vi "AM.vi"() -> ()   [LabVIEW 2015]
uses:
  <vilib>/express/express analysis/Spectral/Block/exnSpectralBlock spectral measurements RMS poly.vi
  <vilib>/express/express analysis/Spectral/Block/exnSpectralBlock spectral measurements RMS DDT.vi
  <vilib>/express/express analysis/Spectral/XNode/ExpressSpectralMeasurementsBlockNode.xnode
panel:
  out "Waveform Graph":dynamicdata(graph)
  out "Message":dynamicdata(graph)
  in  "Carrier Amp":dbl(slide) scale=0.0..10.0
  in  "Message Frequency":dbl(slide) scale=100.0..200.0
  in  "Carrier Frequency":dbl(slide) scale=0.0..10000.0
  out "AM":dynamicdata(graph)
  in  "stop":bool
  in  "m":dbl(slide) scale=0.0..2.0
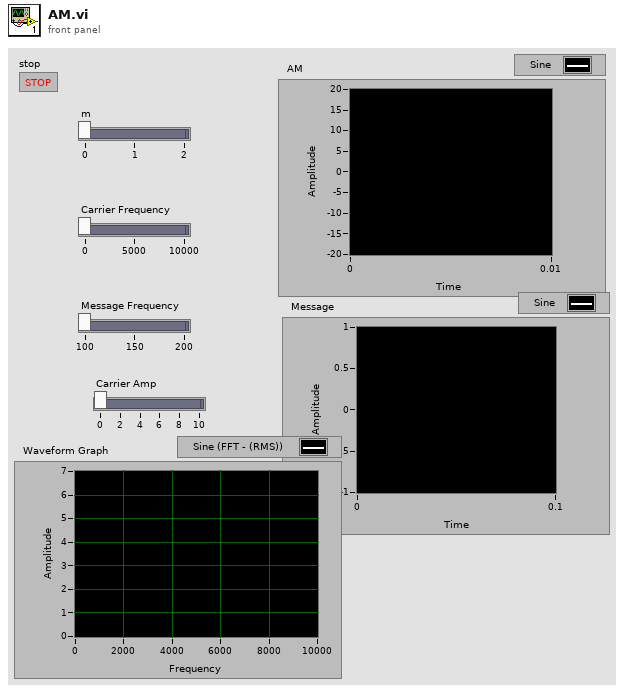
[diagram p1: front panel]
types:
  T1 = cluster{"averaging mode":u16, "weighting mode":u16, "number of averages":u32}
  T2 = cluster{"dB On (F)":bool, "unwrap phase (F)":bool, "convert to degree (F)":bool}
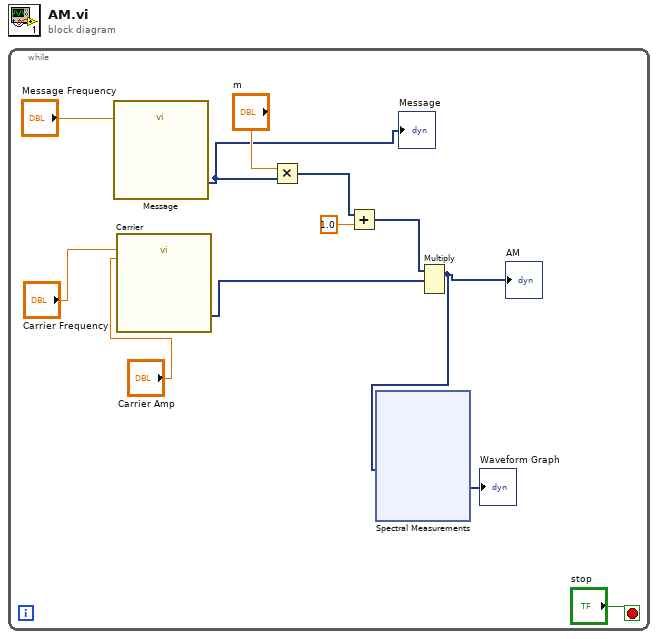
[diagram p0: block diagram]
diagram:
  n1 = while {
    stop <- "stop" stop-if-true
    n2 = call "Message"("Frequency"="Message Frequency") -> ("Sine"=w3:dynamicdata)  [unwired: 13 in, 1 out]
    "Message" <- w3
    n3 = call "Carrier"("Frequency"="Carrier Frequency", "Amplitude"="Carrier Amp") -> ("Sine"=w7:dynamicdata)  [unwired: 12 in, 1 out]
    n4 = Multiply(x="m", y=w3) -> (x*y=w12:dynamicdata)
    n5 = Add(x=w12, y=1.0) -> (x+y=w9:dynamicdata)
    n6 = Multiply(1:w7, 2:w9) -> (0:w2:dynamicdata)  [unwired: 1 in, 1 out]
    "AM" <- w2
    n7 = xnode "Spectral Measurements"("Signals"=w2) -> ("FFT - (RMS)"=→"Waveform Graph":dynamicdata)  [unwired: 1 in, 2 out]
  }
